vi "eventHandler.vi"(8 "error in (no error)":errorcluster, 11 "Compiler in":refnum<class "Compiler.lvclass">) -> (0 "error out":errorcluster, 3 "Compiler out":refnum<class "Compiler.lvclass">)   [LabVIEW 2011, in "Compiler.lvlib" / "Compiler.lvclass"]
uses:
  Compiler.lvclass
  CompiledList/CompiledList.lvclass
  Compiler.lvclass/Compiler.ctl
  Hal/HWController/HWControllerEvents/HWControllerEvents.lvclass
panel:
  out "stop":bool
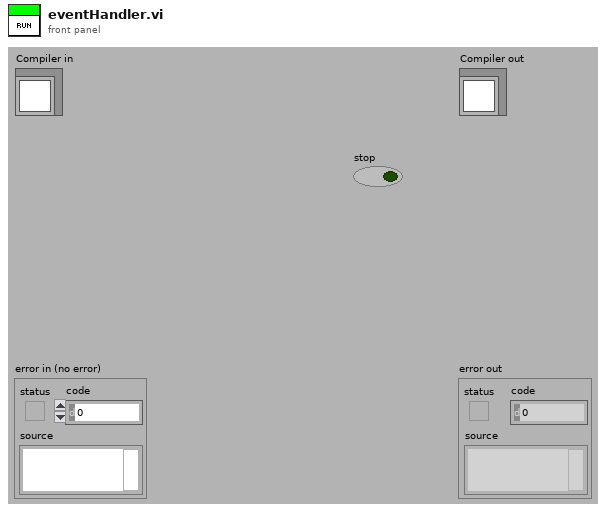
[diagram p1: front panel]
types:
  T1 = cluster{"Compiler in":refnum<class "Compiler.lvclass">, "Compiler.lvlib:CompiledList.lvclass":refnum<class "CompiledList.lvclass">}
  T2 = cluster{"incomingEventTypes":cluster{"start":cluster{"Boolean":bool}, "stop":cluster{"Boolean":bool}, "statusInquiry":cluster{"Boolean":bool}, "configure":cluster{"DPScriptPath":path, "TimeStamp":string, "HWLoop?":bool}, "resetError":cluster{"Boolean":bool}, "resourcesInquiry":cluster{"Boolean":bool}, "reserveResources":cluster{"HWList":string[]}, "initialise":cluster{"HWList":string[]}, "close":cluster{"Boolean":bool}, "resetAllChannels":cluster{"Boolean":bool}, "staticChannelUpdate":cluster{"channel_address":string, "calibratedValue":dbl}, "runScript":cluster{"DPScriptPath":path, "TimeStamp":string, "HWLoop?":bool}, "compilingScript":cluster{"Path":path}, "compiledScript":cluster{"Path":path, "timeCompileAt":string}, "compilerError":cluster{"Path":path}, "configureCompiledScript":cluster{"DPScriptPath":path, "TimeStamp":string, "HWLoop?":bool, "CompiledScript":cluster{"ScriptListCompiler.lvclass":refnum<class "ScriptListCompiler.lvclass">, "aoChannels":refnum<class "AnalogOutput.lvclass">[], "doChannels":refnum<class "DigitalOutput.lvclass">[], "rfChannels":refnum<class "DDSOutput.lvclass">[]}}, "restartCompiler":cluster{"restart":bool}, "staticRfChannelUpdate":cluster{"channel_address":string, "Output":cluster{"Frequency(MHz)":dbl, "Amplitude":dbl, "Phase":dbl, "OutputForm":enum16{"Sine", "Square", "Triangle", "Arbitrary"}}}, "cameraUpdate":cluster{"Camera":string, "Type":string, "settings":path}}, "outgoingEventTypes":cluster{"HWStatus":cluster{"status":enum16{"Ready", "Compiling", "Configured", "Running", "Stopping", "Unresolved Error"}}, "error":cluster{"error out":errorcluster}, "resourcesAvailable":cluster{"availableHWList":string[], "reservedHWList":string[]}, "resourcesReserved":cluster{"reservedHWList":string[]}}}
  T3 = cluster{"Compiler out":refnum<class "Compiler.lvclass">, "CompiledList":refnum<class "CompiledList.lvclass">}
  T4 = enum16{"start", "stop", "statusInquiry", "configure", "resetError", "resourcesInquiry", "reserveResources", "initialise", "resetAllChannels", "staticUpdate", "close", "HWStatus", "error", "resourcesAvailable", "resourcesReserved", "compilerError", "compiledScript", "compilingScript", "runScript", "configureCompiledScript", "restartCompiler", "staticRfChannelUpdate", "cameraUpdate"}
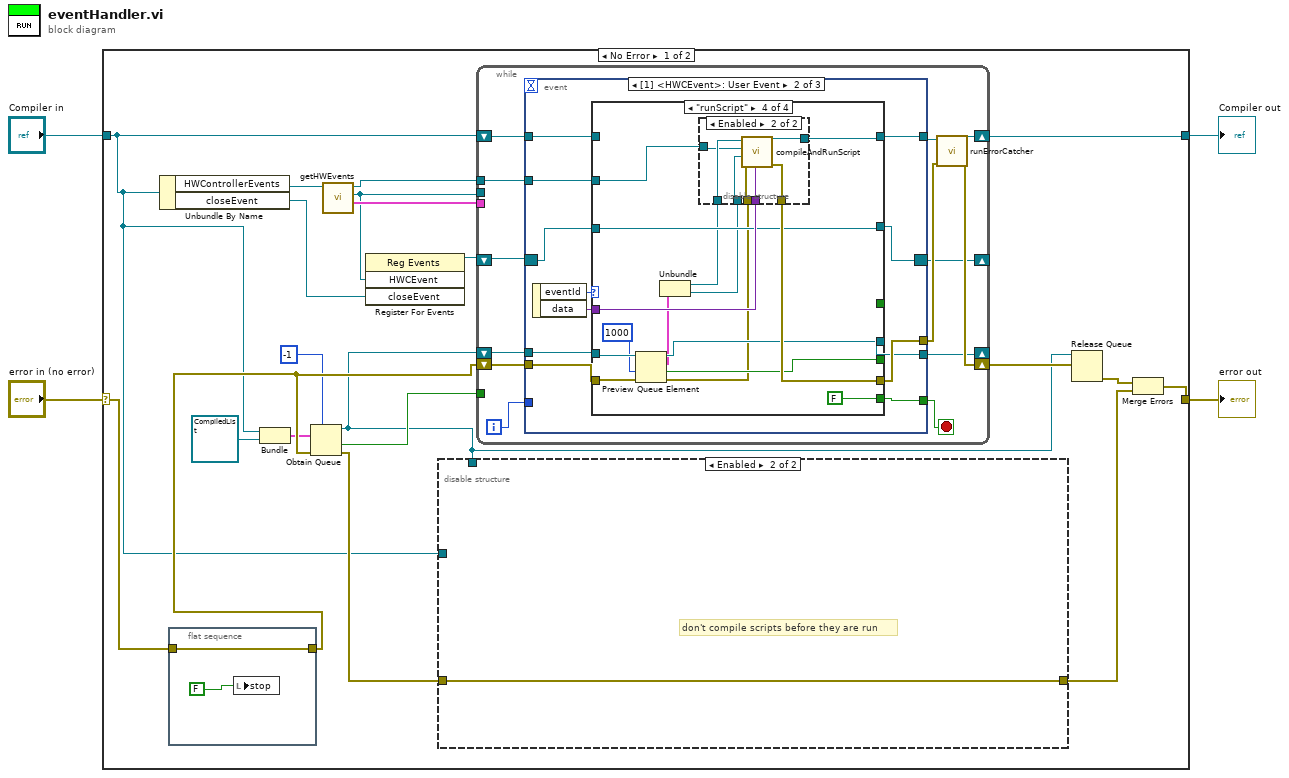
[diagram p0: block diagram]
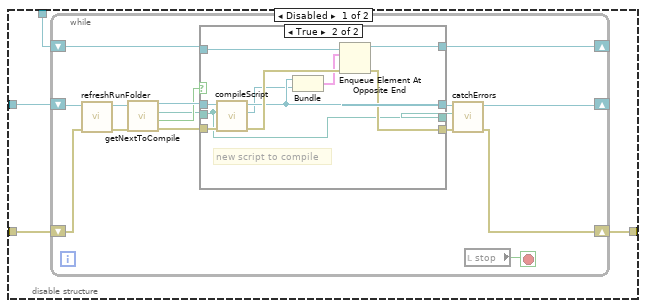
[diagram p2: hidden frame]
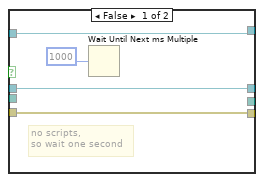
[diagram p3: hidden frame]
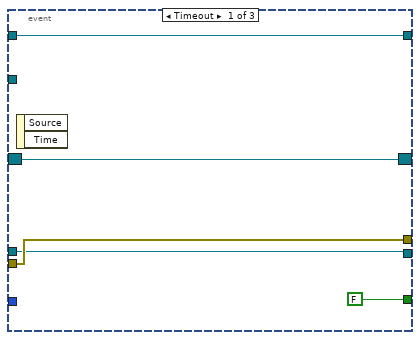
[diagram p4: hidden frame]
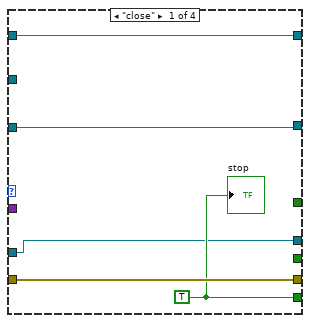
[diagram p5: hidden frame]
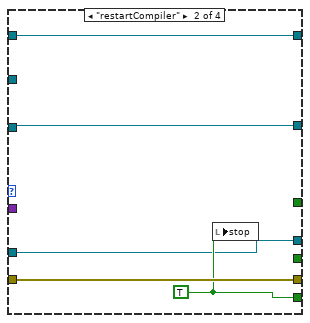
[diagram p6: hidden frame]
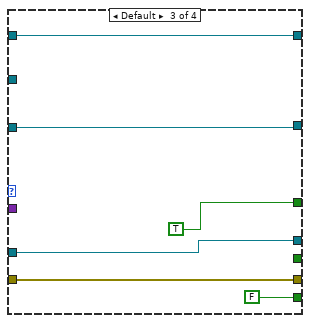
[diagram p7: hidden frame]
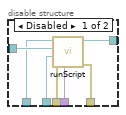
[diagram p8: hidden frame]
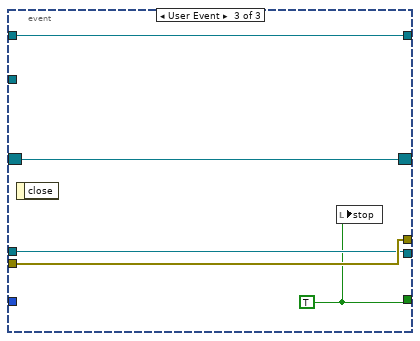
[diagram p9: hidden frame]
diagram:
  n1 = case shown="No Error" "error in (no error)" {
    selector: "error in (no error)" -> [w15 w143]
    tunnel: [w18 w143] -> w3
    tunnel: [w23 w142] -> w1
    tunnel: "Compiler in" -> [w6 w142]
    frame No Error {
      n2 = Unbundle By Name(w6) -> ("HWControllerEvents"=w24:refnum<class "HWControllerEvents.lvclass">, "closeEvent"=w5:refnum<user-event>)
      n3 = flat-sequence {
        tunnel: w15 -> [w60]
        tunnel: [w60] -> w14
        frame #0 {
          n4 = local write "stop"(FALSE) -> ()
        }
      }
      n5 = Bundle("Compiler in"=w6, "Compiler.lvlib:CompiledList.lvclass"=refnum<class "CompiledList.lvclass"> refnum) -> (w7:T1)  [unwired: 1 in]
      n6 = Obtain Queue(max queue size (-1, unlimited)=-1, element data type=w7, error in (no error)=w14) -> (queue out=w9:refnum<queue>, created new?=w10:bool, error out=w19:errorcluster)  [unwired: 2 in]
      n7 = call-dynamic "getHWEvents.vi"("HWControllerEvents in"=w24) -> ("eventDataTypes"=w21:T2, "HWCEvent"=w20:refnum<user-event>, "HWControllerEvents out"=w16:refnum<class "HWControllerEvents.lvclass">)  [unwired: 7 in, 1 out]
      n8 = register-events(w20, w5) -> (reference out=w22:refnum<event-registration>)  [unwired: 2 in, 1 out]
      n9 = disable-structure shown="Enabled" {
        disable-tunnel: w19 -> [w28 w59]
        disable-tunnel: [w27 w59] -> w17
        disable-tunnel: w9 -> [w26 _]
        disable-tunnel: w6 -> [w25 _]
        frame Disabled {
          n10 = while {
            shift-right: [w34] -> w27
            shift-left: w28 -> [w42]
            shift-right: [w31] -> _
            shift-left: w25 -> [w43]
            shift-right: [w29] -> _
            shift-left: w26 -> [w37]
            stop <- w44 stop-if-true
            n11 = call "refreshRunFolder.vi"("error in (no error)"=w42, "Compiler in"=w43) -> ("error out"=w40:errorcluster, "Compiler out"=w41:refnum<class "Compiler.lvclass">)  [unwired: 8 in]
            n12 = call "getNextToCompile.vi"("error in (no error)"=w40, "Compiler in"=w41) -> ("error out"=w39:errorcluster, "newScript?"=w33:bool, "Path"=w32:path, "Compiler out"=w38:refnum<class "Compiler.lvclass">)  [unwired: 6 in]
            n13 = case shown="True" w33 {
              tunnel: w39 -> [w47 w58]
              tunnel: w38 -> [w48 w57]
              tunnel: w37 -> [w45 w55]
              tunnel: [w48 w51] -> w36
              tunnel: [w47 w56] -> w35
              tunnel: w32 -> [_ w53]
              tunnel: [_ w53] -> w30
              tunnel: [w45 w52] -> w29
              frame False {
                # "no scripts,\nso wait one second"
                n14 = Wait Until Next ms Multiple(millisecond multiple=1000) -> ()  [unwired: 1 out]
              }
              frame True {
                # "new script to compile"
                n15 = call "compileScript.vi"("error in (no error)"=w58, "Path"=w53, "Compiler in"=w57) -> ("error out"=w54:errorcluster, "CompiledList"=w50:refnum<class "CompiledList.lvclass">, "Compiler out"=w51:refnum<class "Compiler.lvclass">)  [unwired: 6 in]
                n16 = Bundle("Compiler out"=w51, "CompiledList"=w50) -> (w49:T3)  [unwired: 1 in]
                n17 = Enqueue Element At Opposite End(queue=w55, element=w49, error in (no error)=w54) -> (queue out=w52:refnum<queue>, error out=w56:errorcluster)  [unwired: 1 in, 1 out]
              }
            }
            n18 = call "catchErrors.vi"("error in (no error)"=w35, "Path"=w30, "Compiler in"=w36) -> ("error out"=w34:errorcluster, "Compiler out"=w31:refnum<class "Compiler.lvclass">)  [unwired: 7 in]
            n19 = local read "stop"() -> (w44:bool)
          }
        }
        frame Enabled {
          # "don't compile scripts before they are run"
        }
      }
      n20 = while {
        shift-right: [w67] -> w23
        shift-left: w6 -> [w74]
        tunnel: w20 -> [_]
        tunnel: w21 -> [_]
        shift-right: [w65] -> w13
        shift-left: w14 -> [w72]
        tunnel: w16 -> [w69]
        shift-right: [w63] -> _
        shift-left: w22 -> [w73]
        tunnel: w10 -> [_]
        shift-right: [w62] -> _
        shift-left: w9 -> [w71]
        i -> [w64]
        stop <- w70 stop-if-true
        n21 = event shown="[1] <HWCEvent>: User Event" {
          selector: w73 -> [w77 w83 w138]
          dyn-events: [w77 w82 w138] -> w63
          timeout: _ -> [_ _ _]
          tunnel: w74 -> [w79 w87 w139]
          tunnel: [w79 w88 w139] -> w68
          tunnel: w72 -> [w78 w90 w141]
          tunnel: [w78 w85 w141] -> w66
          tunnel: w71 -> [w75 w89 w140]
          tunnel: [FALSE w84 w137] -> w70
          tunnel: w69 -> [_ w86 _]
          tunnel: w64 -> [_ _ _]
          tunnel: [w75 w80 w140] -> w62
          event Timeout {
            n22 = event-data() -> ()  [unwired: 1 in, 2 out]
          }
          event User Event {
            n23 = event-data() -> ("eventId"=w91:T4, "data"=w81:variant)  [unwired: 1 in]
            n24 = case shown="\"runScript\"" w91 {
              tunnel: w81 -> [_ _ _ w119]
              tunnel: w90 -> [w95 w101 w106 w115]
              tunnel: w89 -> [w92 w97 w102 w116]
              tunnel: [w96 w100 w107 w121] -> w88
              tunnel: w87 -> [w96 w100 w107 _]
              tunnel: w86 -> [_ _ _ w122]
              tunnel: [w95 w101 w106 w120] -> w85
              tunnel: [w94 w98 FALSE FALSE] -> w84
              tunnel: w83 -> [w93 w99 w105 w118]
              tunnel: [w93 w99 w105 w118] -> w82
              tunnel: [_ _ TRUE _] -> _
              tunnel: [_ _ _ w113] -> _
              tunnel: [w92 w97 w102 w112] -> w80
              frame "close" {
                w94 = TRUE
                "stop" <- w94
              }
              frame "restartCompiler" {
                w98 = TRUE
                n25 = local write "stop"(w98) -> ()
              }
              frame Default {
              }
              frame "runScript" {
                n26 = Preview Queue Element(queue=w116, timeout in ms (-1)=1000, error in (no error)=w115) -> (queue out=w112:refnum<queue>, element=w111:T1, timed out?=w113:bool, error out=w108:errorcluster)
                n27 = Unbundle(w111) -> ("Compiler in"=w110:refnum<class "Compiler.lvclass">, "Compiler.lvlib:CompiledList.lvclass"=w109:refnum<class "CompiledList.lvclass">)
                n28 = disable-structure shown="Enabled" {
                  disable-tunnel: w122 -> [w129 w134]
                  disable-tunnel: [w128 w136] -> w121
                  disable-tunnel: [w127 w130] -> w120
                  disable-tunnel: w119 -> [w126 w131]
                  disable-tunnel: w110 -> [w125 w135]
                  disable-tunnel: w109 -> [w124 w133]
                  disable-tunnel: w108 -> [w123 w132]
                  frame Disabled {
                    n29 = call "runScript.vi"("data"=w126, "error in (no error)"=w123, "CompiledList"=w124, "HWControllerEvents in"=w129, "Compiler in"=w125) -> ("error out"=w127:errorcluster, "Compiler out"=w128:refnum<class "Compiler.lvclass">)  [unwired: 5 in]
                  }
                  frame Enabled {
                    n30 = call "compileAndRunScript.vi"("data"=w131, "error in (no error)"=w132, "CompiledList"=w133, "HWControllerEvents in"=w134, "Compiler in"=w135) -> ("error out"=w130:errorcluster, "Compiler out"=w136:refnum<class "Compiler.lvclass">)  [unwired: 5 in]
                  }
                }
              }
            }
          }
          event User Event {
            w137 = TRUE
            n31 = event-data() -> ()  [unwired: 1 in, 1 out]
            n32 = local write "stop"(w137) -> ()
          }
        }
        n33 = call "runErrorCatcher.vi"("error in (no error)"=w66, "Compiler in"=w68) -> ("error out"=w65:errorcluster, "Compiler out"=w67:refnum<class "Compiler.lvclass">)  [unwired: 8 in]
      }
      n34 = Release Queue(queue=w9, error in (no error)=w13) -> (error out=w12:errorcluster)  [unwired: 1 in, 2 out]
      n35 = Merge Errors(w12, w17) -> (w18:errorcluster)
    }
    frame Error {
    }
  }
  "error out" <- w3
  "Compiler out" <- w1
